vi "Include.vi"   [LabVIEW 2017]
uses:
  <resource>/AFDebug/TDM Registration Mode.ctl
  <resource>/AFDebug/This Actor.ctl
  <vilib>/ActorFramework/Message Enqueuer/Message Enqueuer.lvclass
  <resource>/AFDebug/AF Debug.lvlib
panel:
  # "Explicitly include this code to prevent\ncyclic dependency VI Package build problems"
types:
  T1 = typedef "AF Debug.lvlib/This Actor.ctl" = cluster{"Enqueuer":refnum<class "Message Enqueuer.lvclass">, "ID":string, "Alias":string, "Actor Core Name":string, "Details":cluster{"Qualified Name":string, "Caller ID":string}}
  T2 = typedef "AF Debug.lvlib/TDM Registration Mode.ctl" = enum16{"Register TDM", "Get ID", "Get Notifier", "Deregister TDM"}
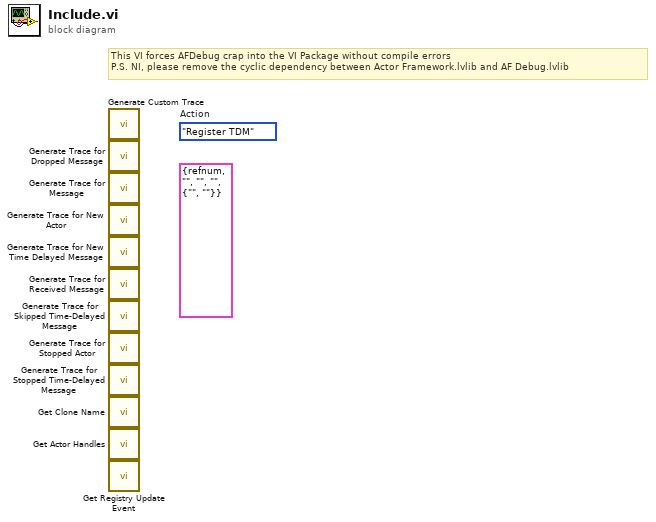
[diagram p0: block diagram]
diagram:
  (unwired) T1 {"Enqueuer"=refnum, "ID"="", "Alias"="", "Actor Core Name"="", "Details"={"Qualified Name"="", "Caller ID"=""}} ("This Actor")
  (unwired) TDM_Registration_Mode."Register TDM"  # Action
  # "This VI forces AFDebug crap into the VI Package without compile errors\nP.S. NI, please remove the cyclic dependency between Actor Framework.lvlib and AF Debug.lvlib"
  n1 = call <resource>:"Generate Custom Trace.vi"() -> ()  [unwired: 12 in]
  n2 = call <resource>:"Generate Trace for Dropped Message.vi"() -> ()  [unwired: 12 in]
  n3 = call <resource>:"Generate Trace for Message.vi"() -> ()  [unwired: 12 in]
  n4 = call <resource>:"Generate Trace for New Actor.vi"() -> ()  [unwired: 12 in]
  n5 = call <resource>:"Generate Trace for New Time Delayed Message.vi"() -> ()  [unwired: 12 in]
  n6 = call <resource>:"Generate Trace for Received Message.vi"() -> ()  [unwired: 12 in]
  n7 = call <resource>:"Generate Trace for Skipped Time-Delayed Message.vi"() -> ()  [unwired: 12 in]
  n8 = call <resource>:"Generate Trace for Stopped Actor.vi"() -> ()  [unwired: 12 in]
  n9 = call <resource>:"Generate Trace for Stopped Time-Delayed Message.vi"() -> ()  [unwired: 12 in]
  n10 = call <resource>:"Get Clone Name.vi"() -> ()  [unwired: 10 in, 2 out]
  n11 = call <resource>:"Get Actor Handles.vi"() -> ()  [unwired: 11 in, 1 out]
  n12 = call <resource>:"Get Registry Update Event.vi"() -> ()  [unwired: 11 in, 1 out]
